vi "string subset.vi"() -> ()   [LabVIEW 2017]
panel:
  out "substring":string
  in  "String":string
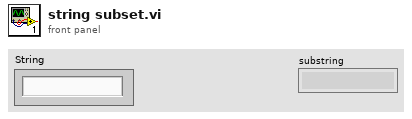
[diagram p1: front panel]
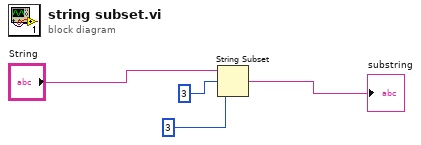
[diagram p0: block diagram]
diagram:
  n1 = String Subset(string="String", offset (0)=3, length (rest)=3 ("length (rest)")) -> (substring=→"substring":string)
